vi "Definy_Earliest_Problem_in_Longest_Track-1.vi"(3 "error IN":errorcluster, 4 "[IN] #of Frames":i32, 5 "[IN] Still connected\ntracks in group":T1) -> (0 "error OUT":errorcluster, 1 "[OUT] # of Longest track\nInside the Group of Tracks":i32, 2 "[OUT] Index of Problem\nPoint Inside Track":i32)   [LabVIEW 2013]
doc: "Subprogram: \n- defines the earliest problem point between all tracks;\n- after defines the longest track containing this problem point"
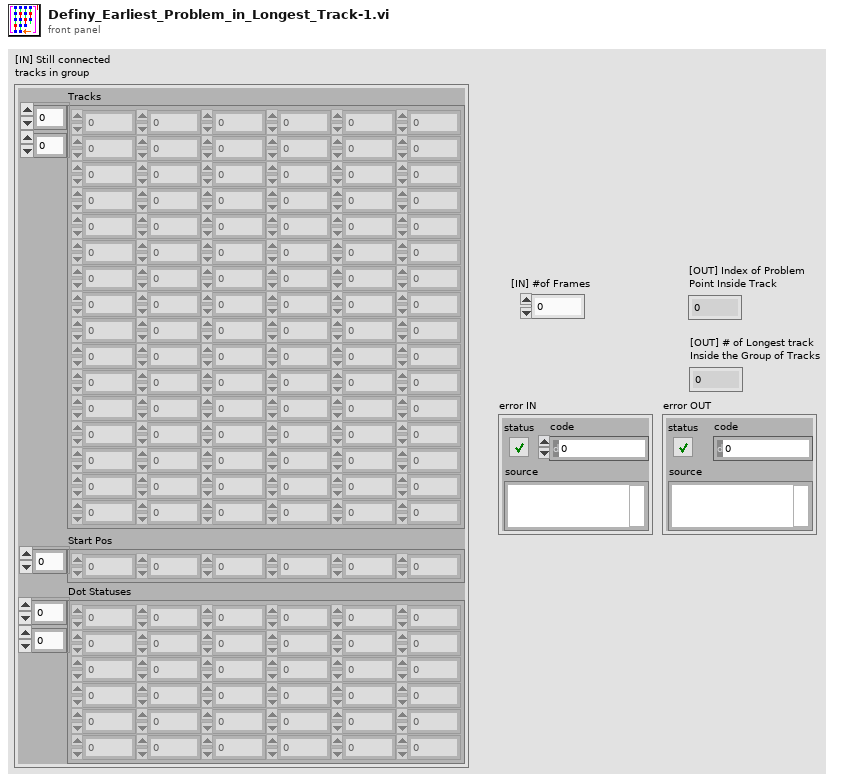
[diagram p1: front panel]
types:
  T1 = cluster{"Tracks":dbl[][], "Start Pos":i32[], "Dot Statuses":i16[][]}
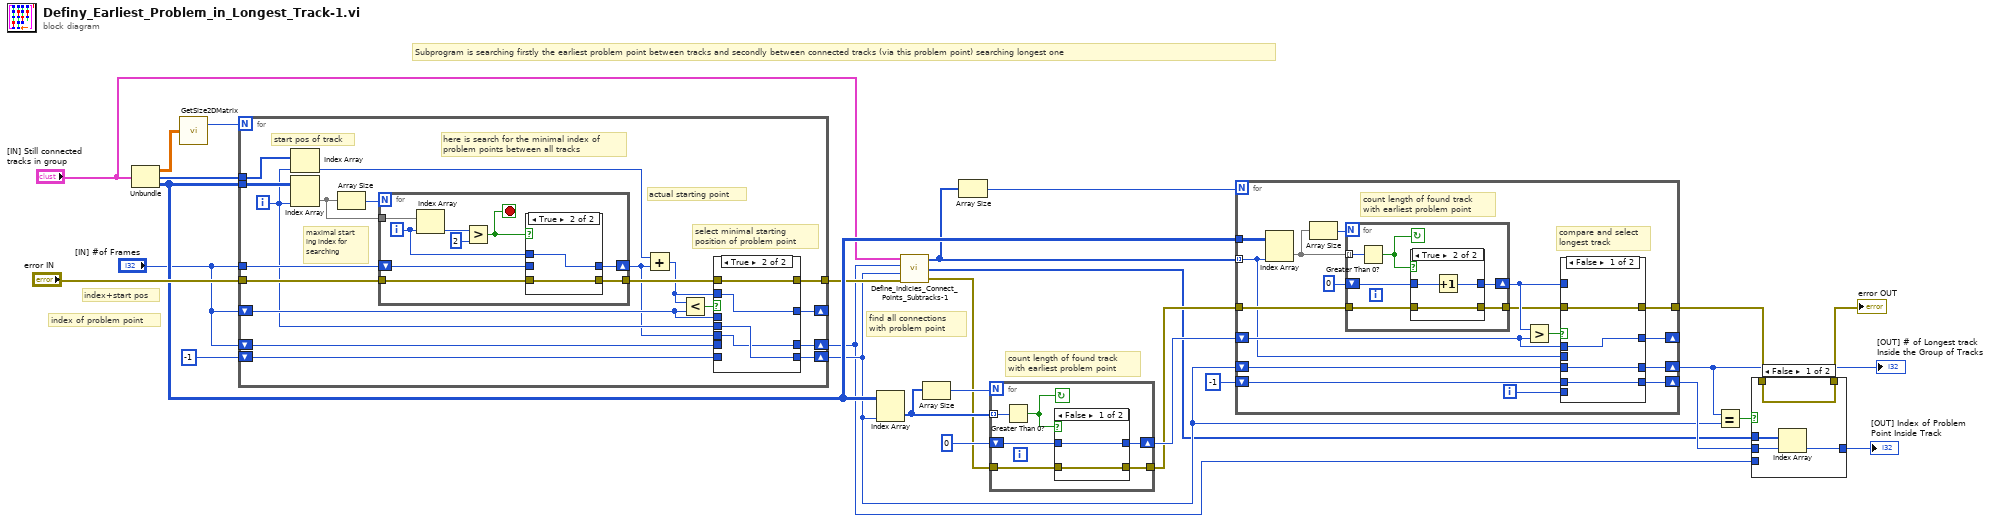
[diagram p0: block diagram]
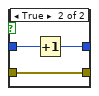
[diagram p3: hidden frame]
diagram:
  # "index of problem point"
  # "index+start pos"
  # "count length of found track\nwith earliest problem point"
  # "find all connections \nwith problem point"
  # "Subprogram is searching firstly the earliest problem point between tracks and secondly between connected tracks (via this problem point) searching longest one"
  n1 = Unbundle("[IN] Still connected\ntracks in group") -> ("Tracks"=w27:dbl[][], "Start Pos"=w26:i32[], "Dot Statuses"=w18:i16[][])
  n2 = call "GetSize2DMatrix.vi"("Array IN (2D)"=w27) -> ("# Cols"=w25:i32)  [unwired: 1 out]
  n3 = for {
    N: w25 -> [_]
    tunnel: w18 -> [w46]
    tunnel: w26 -> [w45]
    shift-right: [w39] -> _
    shift-left: "[IN] #of Frames" -> [w40]
    tunnel: "[IN] #of Frames" -> [w42]
    tunnel: "error IN" -> [w38]
    tunnel: [w36] -> w7
    shift-right: [w33] -> w6
    shift-left: -1 ("# Cols") -> [w35]
    shift-right: [w29] -> w5
    shift-left: "[IN] #of Frames" -> [w30]
    i -> [w34]
    # "actual starting point"
    # "here is search for the minimal index of \nproblem points between all tracks"
    # "select minimal starting \nposition of problem point"
    # "maximal start\ning index for\nsearching"
    # "start pos of track"
    n4 = Index Array(array=w45, index=w34) -> (element=w32:i32)
    n5 = Index Array(array=w46, index (col)=w34) -> (element=w43:i16[])  [unwired: 1 in]
    n6 = Array Size(array=w43) -> (size(s)=w44:i32)
    n7 = for {
      N: w44 -> [_]
      tunnel: w43 -> [w63]
      shift-right: [w57] -> w28
      shift-left: w42 -> [w59]
      tunnel: w38 -> [w56]
      tunnel: [w55] -> w37
      i -> [w58]
      stop <- w60 stop-if-true
      n8 = Index Array(array=w63, index=w58) -> (element=w62:i16)
      n9 = Greater?(x=w62, y=i16 2) -> (0:w60:bool)
      n10 = case shown="True" w60 {
        tunnel: w59 -> [w65 _]
        tunnel: w58 -> [_ w67]
        tunnel: [w65 w67] -> w57
        tunnel: w56 -> [w64 w66]
        tunnel: [w64 w66] -> w55
        frame False {
        }
        frame True {
        }
      }
    }
    n11 = Add(x=w32, y=w28) -> (x+y=w31:i32)
    n12 = Less?(x=w31, y=w40) -> (x < y?=w41:bool)
    n13 = case shown="True" w41 {
      tunnel: w40 -> [w50 _]
      tunnel: [w50 w54] -> w39
      tunnel: w31 -> [_ w54]
      tunnel: w37 -> [w49 w53]
      tunnel: [w49 w53] -> w36
      tunnel: w35 -> [w48 _]
      tunnel: w34 -> [_ w52]
      tunnel: [w48 w52] -> w33
      tunnel: w30 -> [w47 _]
      tunnel: [w47 w51] -> w29
      tunnel: w28 -> [_ w51]
      frame False {
        # "index"
        # "index+start\npos"
      }
      frame True {
      }
    }
  }
  n14 = Index Array(array=w18, index (col)=w6) -> (element=w20:i16[])  [unwired: 1 in]
  n15 = call "Define_Indicies_Connect_Points_Subtracks-1.vi"("error IN"=w7, "[IN] Index of track with\n(problem displacement)"=w6, "[IN] Index of problem\ndisplacement inside track"=w5, "[IN] Track group"="[IN] Still connected\ntracks in group") -> ("error OUT"=w1:errorcluster, "[OUT] Index of \nconnected dots\ninside the track"=w2:i32[], "[OUT] Index of connected\ntracks with problem dot"=w3:i32[])
  n16 = Array Size(array=w20) -> (size(s)=w21:i32)
  n17 = Array Size(array=w3) -> (size(s)=w22:i32)
  n18 = for {
    N: w21 -> [_]
    tunnel: w20 -> [w73] mode=indexing
    shift-right: [w70] -> w17
    shift-left: 0 -> [w71]
    tunnel: w1 -> [w69]
    tunnel: [w68] -> w16
    stop <- w72 continue-if-true
    n19 = Greater Than 0?(x=w73) -> (x > 0?=w72:bool)
    n20 = case shown="False" w72 {
      tunnel: w71 -> [w75 w78]
      tunnel: [w75 w77] -> w70
      tunnel: w69 -> [w74 w76]
      tunnel: [w74 w76] -> w68
      frame False {
      }
      frame True {
        n21 = Increment(x=w78) -> (x+1=w77:i32)
      }
    }
  }
  n22 = for {
    N: w22 -> [_]
    tunnel: w3 -> [w83] mode=indexing
    tunnel: w18 -> [w92]
    tunnel: w16 -> [w91]
    shift-right: [w86] -> _
    shift-left: w17 -> [w88]
    shift-right: [w84] -> w10
    shift-left: w6 -> [w85]
    tunnel: [w82] -> w13
    shift-right: [w80] -> w8
    shift-left: -1 -> [w81]
    i -> [w79]
    # "compare and select\nlongest track"
    # "count length of found track\nwith earliest problem point"
    n23 = Index Array(array=w92, index (col)=w83) -> (element=w94:i16[])  [unwired: 1 in]
    n24 = Array Size(array=w94) -> (size(s)=w95:i32)
    n25 = for {
      N: w95 -> [_]
      tunnel: w94 -> [w109] mode=indexing
      shift-right: [w106] -> w89
      shift-left: 0 -> [w107]
      tunnel: w91 -> [w105]
      tunnel: [w104] -> w87
      stop <- w108 continue-if-true
      n26 = Greater Than 0?(x=w109) -> (x > 0?=w108:bool)
      n27 = case shown="True" w108 {
        tunnel: w107 -> [w111 w114]
        tunnel: [w111 w113] -> w106
        tunnel: w105 -> [w110 w112]
        tunnel: [w110 w112] -> w104
        frame False {
        }
        frame True {
          n28 = Increment(x=w114) -> (x+1=w113:i32)
        }
      }
    }
    n29 = Greater?(x=w89, y=w88) -> (0:w90:bool)
    n30 = case shown="False" w90 {
      tunnel: w89 -> [_ w103]
      tunnel: w88 -> [w99 _]
      tunnel: w87 -> [w97 w101]
      tunnel: [w99 w103] -> w86
      tunnel: w85 -> [w98 _]
      tunnel: [w98 w102] -> w84
      tunnel: w83 -> [_ w102]
      tunnel: [w97 w101] -> w82
      tunnel: w81 -> [w96 _]
      tunnel: [w96 w100] -> w80
      tunnel: w79 -> [_ w100]
      frame False {
      }
      frame True {
      }
    }
  }
  "[OUT] # of Longest track\nInside the Group of Tracks" <- w10
  n31 = Equal?(x=w10, y=w6) -> (x = y?=w14:bool)
  n32 = case shown="False" w14 {
    tunnel: w13 -> [w118 w120]
    tunnel: [w118 w120] -> w12
    tunnel: w2 -> [w117 _]
    tunnel: w5 -> [_ w119]
    tunnel: [w115 w119] -> w11
    tunnel: w8 -> [w116 _]
    frame False {
      n33 = Index Array(array=w117, index=w116) -> (element=w115:i32)
    }
    frame True {
    }
  }
  "error OUT" <- w12
  "[OUT] Index of Problem\nPoint Inside Track" <- w11
